vi "GetTestSuites.vi"(8 "error in (no error)":errorcluster) -> (0 "error out":errorcluster, 2 "Tests":refnum<class "Test.lvclass">[](array[class]))   [LabVIEW 2019, in "TestExplorer.lvlib"]
doc: "Returns a list of test suites from the current project.\n\n- Test libraries must be at the top-level inside the project (sublibraries will be ignored)\n- Test library names must end with \"Test.lvlib\""
uses:
  TestExplorer.lvlib
  Test/Test.lvclass
  TestBuilder/TestBuilder.lvclass
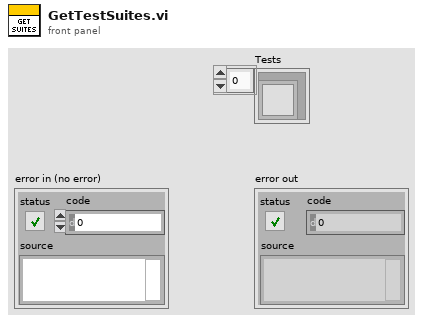
[diagram p1: front panel]
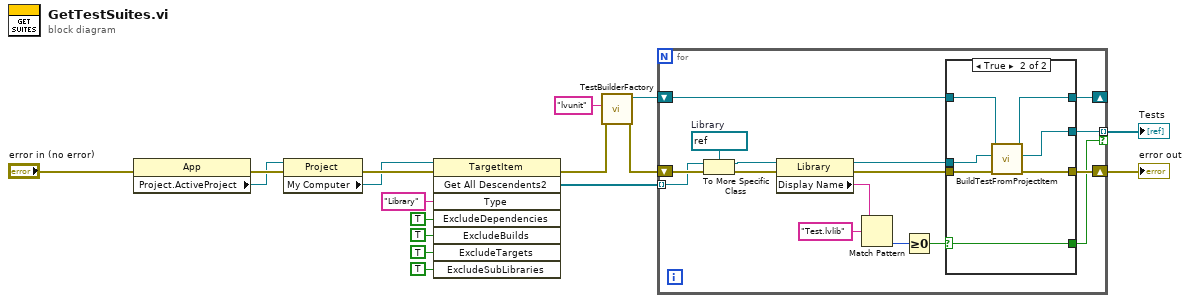
[diagram p0: block diagram]
diagram:
  n1 = property class="App"(error in="error in (no error)") -> (error out=w7:errorcluster, "Project.ActiveProject"=w5:refnum<vi>)  [unwired: 1 in, 1 out]
  n2 = property class="Project"(reference=w5, error in=w7) -> (error out=w17:errorcluster, "My Computer"=w10:refnum<vi>)  [unwired: 1 out]
  n3 = invoke class="TargetItem" method="Get All Descendents2"(reference=w10, error in=w17, "Type"="Library", "ExcludeDependencies"=TRUE, "ExcludeBuilds"=TRUE, "ExcludeTargets"=TRUE, "ExcludeSubLibraries"=TRUE) -> (error out=w3:errorcluster, "Get All Descendents2"=w12:refnum<vi>[])  [unwired: 1 in, 6 out]
  n4 = call "TestBuilderFactory.vi"("error in (no error)"=w3, "Name"="lvunit") -> ("error out"=w2:errorcluster, "Test Builder"=w4:refnum<class "TestBuilder.lvclass">)  [unwired: 8 in]
  n5 = for {
    tunnel: w12 -> [w28] mode=indexing
    shift-right: [w24] -> w9
    shift-left: w2 -> [w30]
    tunnel: [w22] -> w8 mode=indexing if=w21
    shift-right: [w19] -> _
    shift-left: w4 -> [w18]
    w27 = refnum<vi> refnum  # Library
    n6 = To More Specific Class(target class=w27, reference=w28, error in=w30) -> (specific class reference=w26:refnum<vi>, error out=w29:errorcluster)
    n7 = property class="Library"(reference=w26, error in=w29) -> (reference out=w20:refnum<vi>, error out=w25:errorcluster, "Display Name"=w31:string)
    n8 = Match Pattern(string=w31, regular expression="Test.lvlib") -> (offset past match=w32:i32)  [unwired: 1 in, 3 out]
    n9 = Greater Or Equal To 0?(x=w32) -> (x >= 0?=w23:bool)
    n10 = case shown="True" w23 {
      selector: w23 -> [w35 w43]
      tunnel: w25 -> [w36 w42]
      tunnel: [w36 w40] -> w24
      tunnel: [_ w39] -> w22
      tunnel: [w35 w43] -> w21
      tunnel: w20 -> [_ w41]
      tunnel: [w34 w38] -> w19
      tunnel: w18 -> [w34 w37]
      frame False {
      }
      frame True {
        n11 = call-dynamic "BuildTestFromProjectItem.vi"("error in (no error)"=w42, "ProjectItem Refnum"=w41, "TestBuilder in"=w37) -> ("error out"=w40:errorcluster, "Test"=w39:refnum<class "Test.lvclass">, "TestBuilder out"=w38:refnum<class "TestBuilder.lvclass">)  [unwired: 6 in]
      }
    }
  }
  "error out" <- w9
  "Tests" <- w8
